vi "06c-arrays.vi"() -> ()   [LabVIEW 2018, in "LV2Julia_examples.lvlib"]
uses:
  LV2Julia_examples.lvlib
  LV2Julia_core/VIs/Server or client state.ctl
  statistics.ctl
  LV2Julia_core/VIs/Commands.ctl
  LV2Julia_core/VIs/ZMQ timeouts.ctl
  0d29fc62-3d1d-4713-a954-9c9e873b3633.vi
  aea790a6-a42b-4eb0-905f-734239196901.vi
  72a46192-383e-4ee5-9465-71670922b82a.vi
  ef5408d4-6538-41d1-b296-fda05a71e4b0.vi
  b8d67b76-17b0-4ad8-b521-2f6549c52c10.vi
  e4efb182-1b04-4d49-96a3-1defebd055ea.vi
  ef458cb0-9ca2-4aa9-bd1e-ad103f8bb0c0.vi
  9df197b6-2616-4b86-abf4-a70e9215d122.vi
  28751878-cf8c-4743-a8b0-c60d78ce5b36.vi
  c328879f-33e1-4261-a6aa-c93c9ebac265.vi
  0d29fc62-3d1d-4713-a954-9c9e873b3633.vi/8ee49078-a04b-40cf-aceb-de90d52f19ef.vi
  aea790a6-a42b-4eb0-905f-734239196901.vi/353007a7-a356-474a-8eac-0d4386ef6058.vi
  72a46192-383e-4ee5-9465-71670922b82a.vi/fff5125a-c1cf-426f-b211-502a59584787.vi
  ef5408d4-6538-41d1-b296-fda05a71e4b0.vi/38f70dbe-b881-407f-ae9e-ee3877922e21.vi
  b8d67b76-17b0-4ad8-b521-2f6549c52c10.vi/b12f13d0-0083-497f-bd73-45587d52367a.vi
  e4efb182-1b04-4d49-96a3-1defebd055ea.vi/02b7e865-0b9c-4fe2-9305-325b12209529.vi
  e4efb182-1b04-4d49-96a3-1defebd055ea.vi/bae9804c-4c06-4ca2-bba6-84ede4188db3.vi
  ef458cb0-9ca2-4aa9-bd1e-ad103f8bb0c0.vi/e8b90c0a-49a5-4093-b01b-c91da666bc06.vi
  9df197b6-2616-4b86-abf4-a70e9215d122.vi/e68dc8aa-e036-44d5-82eb-549111025a95.vi
  28751878-cf8c-4743-a8b0-c60d78ce5b36.vi/748d803b-9eab-4607-80f6-e121fa062447.vi
  c328879f-33e1-4261-a6aa-c93c9ebac265.vi/2931e3ef-e8d8-47e5-81f6-8bdf84f9b635.vi
  c328879f-33e1-4261-a6aa-c93c9ebac265.vi/2af4d478-d114-4323-a1a4-ea8d6e36c34a.vi
  72a46192-383e-4ee5-9465-71670922b82a.vi/fff5125a-c1cf-426f-b211-502a59584787.vi/7beb9e5a-56af-4202-a395-c072f8f6a12a.vi
  ef5408d4-6538-41d1-b296-fda05a71e4b0.vi/38f70dbe-b881-407f-ae9e-ee3877922e21.vi/706c9d30-0200-4f77-8390-edf6001941d7.vi
  b8d67b76-17b0-4ad8-b521-2f6549c52c10.vi/b12f13d0-0083-497f-bd73-45587d52367a.vi/c2cf4afe-14de-4a7c-a038-eb38a913b356.vi
  b8d67b76-17b0-4ad8-b521-2f6549c52c10.vi/b12f13d0-0083-497f-bd73-45587d52367a.vi/7452286d-6709-42b4-a933-263885f1ef29.vi
  b8d67b76-17b0-4ad8-b521-2f6549c52c10.vi/b12f13d0-0083-497f-bd73-45587d52367a.vi/11fbbbb9-4c5b-4442-95b0-52ac404484f0.vi
  e4efb182-1b04-4d49-96a3-1defebd055ea.vi/02b7e865-0b9c-4fe2-9305-325b12209529.vi/2a070854-1c7d-4d64-a736-cedc11a7f453.vi
  e4efb182-1b04-4d49-96a3-1defebd055ea.vi/02b7e865-0b9c-4fe2-9305-325b12209529.vi/ce6c50d9-0aec-4ce5-9563-f5a1f3a5f606.vi
  9df197b6-2616-4b86-abf4-a70e9215d122.vi/e68dc8aa-e036-44d5-82eb-549111025a95.vi/f53deb3e-8950-4786-9e71-9c0eddecade7.vi
  28751878-cf8c-4743-a8b0-c60d78ce5b36.vi/748d803b-9eab-4607-80f6-e121fa062447.vi/dbe84567-7ef4-485c-b551-38ee1d34b483.vi
  28751878-cf8c-4743-a8b0-c60d78ce5b36.vi/748d803b-9eab-4607-80f6-e121fa062447.vi/ee701064-8ef7-4cb3-acd2-d09a2ca746d4.vi
  28751878-cf8c-4743-a8b0-c60d78ce5b36.vi/748d803b-9eab-4607-80f6-e121fa062447.vi/44459596-931b-4795-b592-1aeed408307a.vi
  c328879f-33e1-4261-a6aa-c93c9ebac265.vi/2931e3ef-e8d8-47e5-81f6-8bdf84f9b635.vi/73e3ce9d-932f-4e3b-9fa0-1650b3f4c481.vi
  c328879f-33e1-4261-a6aa-c93c9ebac265.vi/2931e3ef-e8d8-47e5-81f6-8bdf84f9b635.vi/5f9fe6bb-1a1a-4cc4-87dc-92c210ea0b8d.vi
  72a46192-383e-4ee5-9465-71670922b82a.vi/fff5125a-c1cf-426f-b211-502a59584787.vi/7beb9e5a-56af-4202-a395-c072f8f6a12a.vi/02adab04-5a86-4a97-93e3-27cb657de44c.vi
  ef5408d4-6538-41d1-b296-fda05a71e4b0.vi/38f70dbe-b881-407f-ae9e-ee3877922e21.vi/706c9d30-0200-4f77-8390-edf6001941d7.vi/2e058e94-5032-4d2b-9353-3bd516f74917.vi
  e4efb182-1b04-4d49-96a3-1defebd055ea.vi/02b7e865-0b9c-4fe2-9305-325b12209529.vi/2a070854-1c7d-4d64-a736-cedc11a7f453.vi/5828844a-d6ce-4aa0-80c3-aaf83f58a5bd.vi
  9df197b6-2616-4b86-abf4-a70e9215d122.vi/e68dc8aa-e036-44d5-82eb-549111025a95.vi/f53deb3e-8950-4786-9e71-9c0eddecade7.vi/7afa4ec8-e56f-4750-a570-ce5d96af2d90.vi
  c328879f-33e1-4261-a6aa-c93c9ebac265.vi/2931e3ef-e8d8-47e5-81f6-8bdf84f9b635.vi/73e3ce9d-932f-4e3b-9fa0-1650b3f4c481.vi/979e58dc-c8d9-47e6-a478-8cf7a84a3445.vi
  LV2Julia_core/VIs/check ID validity.vi
  LV2Julia_core/VIs/bindata_descr to JSON.vi
  LV2Julia_core/VIs/check cluster field names.vi
  LV2Julia_core/VIs/concat JSON.vi
  LV2Julia_core/VIs/build request.vi
  LV2Julia_core/VIs/Parse server response.vi
  LV2Julia_core/VIs/log jl exceptions.vi
  <vilib>/Utility/error.llb/Error Cluster From Error Code.vi
  LV2Julia_core/LV2Julia_core.lvlib
panel:
  out "Statistics 1":T1={"size "=0, "mean"=nan, "median"=nan, "min"=nan, "max"=nan} caption="Statistics (ms)" {"min" format="%#.1f"; "max" format="%#.1f"; "median" format="%.1f"; "mean" format="%.1f"}
  in  "max size 1":i32=20 caption="sample max"
  out "Statistics 2":T1={"size "=0, "mean"=nan, "median"=nan, "min"=nan, "max"=nan} caption="Statistics (ms)" {"min" format="%#.1f"; "max" format="%#.1f"; "median" format="%.1f"; "mean" format="%.1f"}
  in  "max size 2":i32=20 caption="sample max"
  out "error info 2":string
  out "call duration (ms) 2":dbl format="%#.3f"
  in  "N - arr size 2":u16=4
  out "Input Matrix (NxN)2":dbl[][](array[numeric])=[[1.0, 0.0, 5.0], [4.0, 2.0, 1.0], [2.0, 2.0, 3.0]] format="%#.4g"
  in  "paus2":bool
  out "current error 2":errorcluster
  out "error info 1":string
  out "call duration (ms) 1":dbl format="%#.3f"
  in  "N - arr size 1":u16=4
  out "Solution Vector":dbl[](array[numeric]) format="%.4f"
  out "Known Vector":dbl[](array[numeric])=[22.0, 14.0, 18.0] format="%#.4g"
  out "Input Matrix (NxN) 1":dbl[][](array[numeric])=[[1.0, 0.0, 5.0], [4.0, 2.0, 1.0], [2.0, 2.0, 3.0]] format="%#.4g"
  in  "paus1":bool
  out "current error 1":errorcluster
  out "Eigenvalues":cdb[](array[numeric]) format="%.2f"
  out "final error":errorcluster
  in  "stop":bool
  out "ZMQ timeout":bool
  out "Jl Server state":T2
  # "Concurrent access to Julia server: Solving a system of linear equations in one loop, and computing eigenvalues in another one."
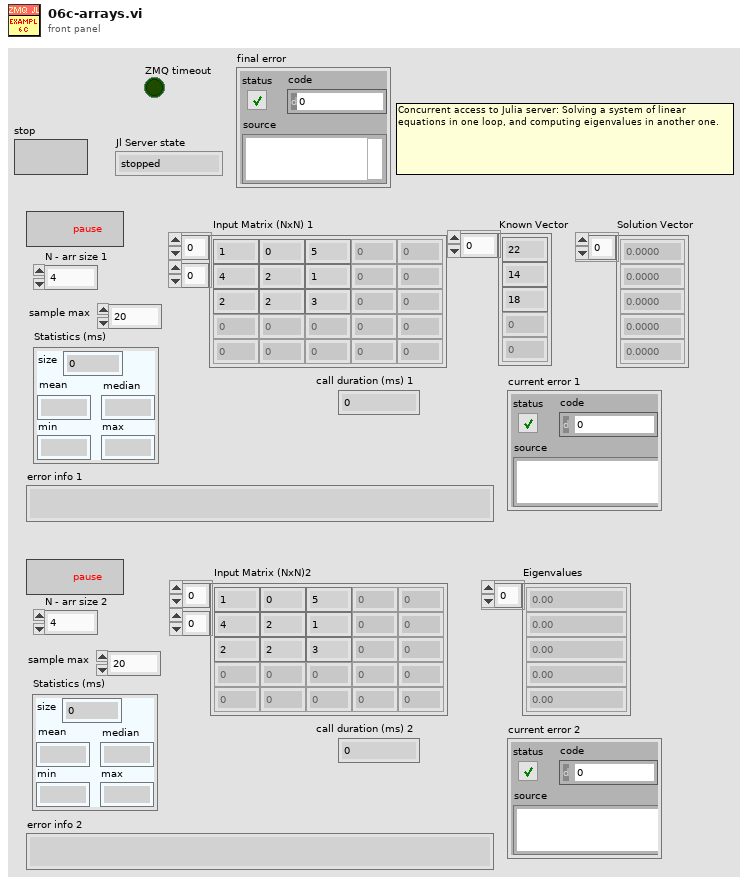
[diagram p1: front panel]
types:
  T1 = typedef "LV2Julia_examples.lvlib/statistics.ctl" = cluster{"size ":u32, "mean":dbl, "median":dbl, "min":dbl, "max":dbl}
  T2 = typedef "LV2Julia_core.lvlib/Server or client state.ctl" = enum16{"stopped", "running", "unknown"}
  T3 = typedef "LV2Julia_core.lvlib/ZMQ timeouts.ctl" = cluster{"SNDTIMEO":i32, "RCVTIMEO":i32}
  T4 = typedef "LV2Julia_core.lvlib/Commands.ctl" = enum16{"Start Jl-server & Init LV-client", "Send request & Get response ", "Stop Jl-server & Cleanup LV-client", "Cleanup LV-client", "Start Jl-server", "Stop Jl-server", "Init LV-Client", "Cleanup LV-Client", "(not allowed)", "Set LV Client state", "Set Jl Server state", "set ZMQ timeout", "read ZMQ timeout", "read-out state"}
  T5 = typedef "LV2Julia_core.lvlib/Bindata&description.ctl" = cluster{"bindata_descr":T6[], "bindata":u8[]}
  T6 = typedef "LV2Julia_core.lvlib/Bindata description.ctl" = cluster{"nofbytes":i32, "numtype":string, "start":i32, "arrdims":i32[], "kwarg_name":string, "category":string}
  T7 = typedef "LV2Julia_core.lvlib/detailed error info.ctl" = cluster{"exception_or_info":string, "trace":T8[]}
  T8 = typedef "LV2Julia_core.lvlib/StackFrame.ctl" = cluster{"frame_summary":string, "func":string, "linfo":string, "file":string, "line":i32, "pointer":u64, "from_c":bool, "inlined":bool}
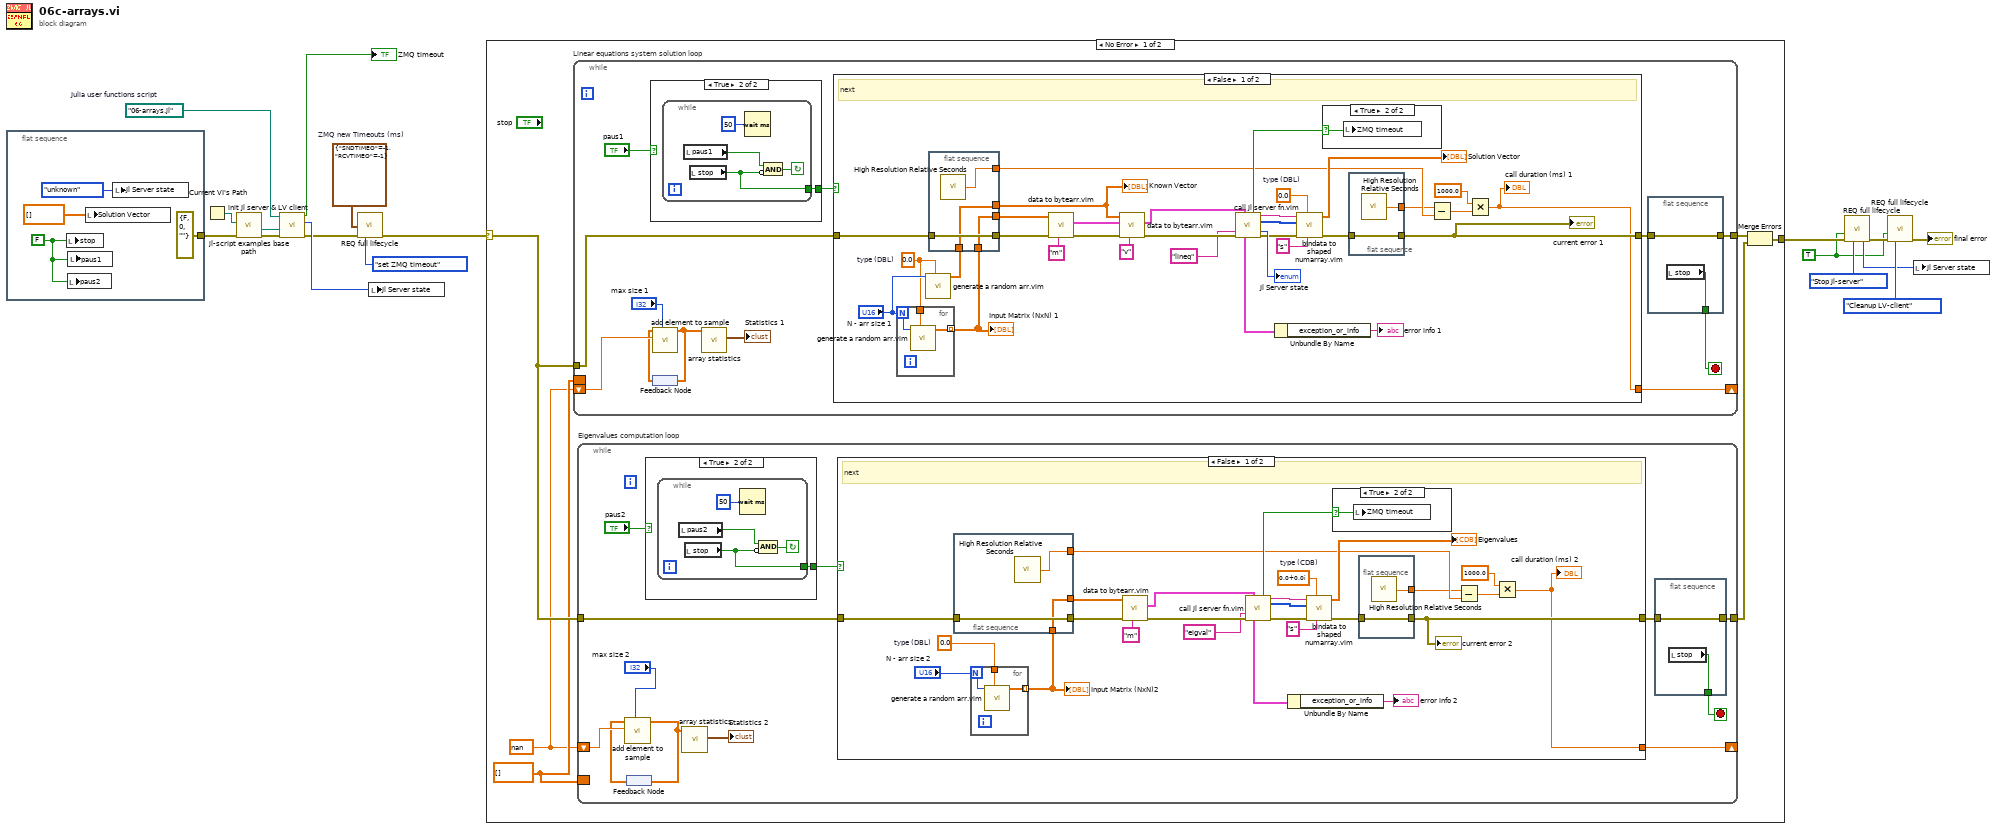
[diagram p0: block diagram]
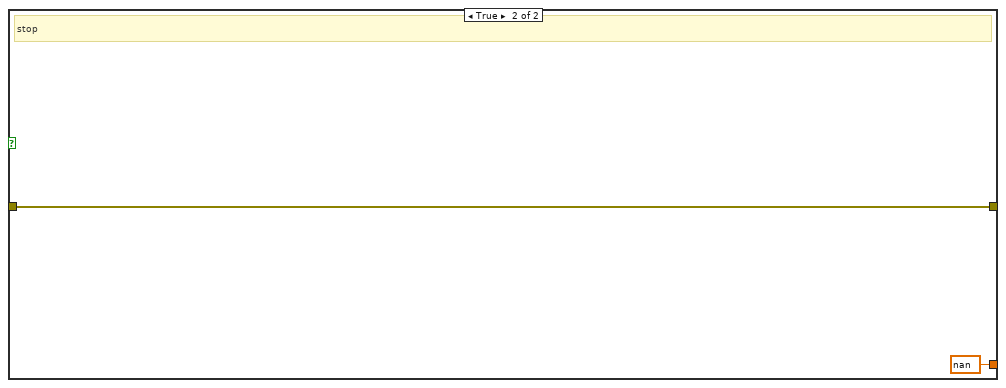
[diagram p4: hidden frame]
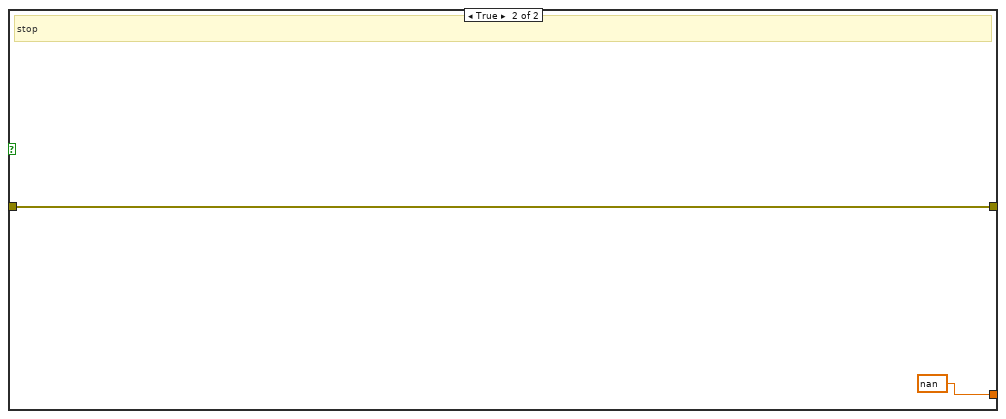
[diagram p7: hidden frame]
diagram:
  w9 = T3 {"SNDTIMEO"=-1, "RCVTIMEO"=-1}  # ZMQ new Timeouts (ms)
  w8 = path "06-arrays.jl"  # Julia user functions script
  w12 = TRUE ("Force command")
  n1 = flat-sequence {
    tunnel: [errorcluster {"status"=FALSE, "code"=0, "source"=""} ("error in (no error)")] -> w1
    frame #0 {
      w19 = FALSE ("stop")
      n2 = local write "stop"(w19) -> ()
      n3 = local write "paus2"(w19) -> ()
      n4 = local write "paus1"(w19) -> ()
      n5 = local write "Solution Vector"(dbl[] [] ("Server response")) -> ()
      n6 = local write "Jl Server state"(Server_or_client_state."unknown" ("Jl Server state out")) -> ()
    }
  }
  n7 = Current VI's Path() -> (path=w4:path)
  n8 = call "jl-script examples base path.vi"("error in (no error)"=w1, "calling example VI path"=w4) -> ("error out"=w3:errorcluster, "jl-script-examples base path"=w2:path)  [unwired: 8 in]
  n9 = call "init Jl server & LV client.vi"("error in (no error)"=w3, "Base path (not a path)"=w2, "Julia user functions script"=w8) -> ("error out"=w5:errorcluster, "Jl Server state out"=w6:T2, "timeout?"=→"ZMQ timeout":bool)  [unwired: 6 in]
  n10 = call "REQ full lifecycle.vi"("ZMQ new Timeouts in"=w9, "error in"=w5, "command"=Commands."set ZMQ timeout") -> ("error out"=w11:errorcluster)  [unwired: 6 in, 6 out]
  n11 = local write "Jl Server state"(w6) -> ()
  n12 = case shown="No Error" w11 {
    selector: w11 -> [w25 w148]
    tunnel: [w27 w148] -> w18
    frame No Error {
      w24 = dbl[] []
      w23 = nan
      n13 = while "Linear equations system solution loop" {
        tunnel: w25 -> [w91]
        tunnel: [w95] -> w28
        shift-right: [w90] -> _
        shift-left: w23 -> [w89]
        border: w24 -> [_]
        stop <- w94 stop-if-true
        n14 = case shown="True" "paus1" {
          tunnel: [_ w97] -> w93
          frame False {
          }
          frame True {
            n15 = while {
              tunnel: [w98] -> w97
              stop <- w99 continue-if-true
              n16 = local read "paus1"() -> (w100:bool)
              n17 = local read "stop"() -> (w98:bool)
              n18 = Wait (ms)(milliseconds to wait=u32 50) -> ()  [unwired: 1 out]
              n19 = Compound Arithmetic op=AND(w100, invert w98) -> (w99:bool)
            }
          }
        }
        n20 = feedback #1() -> (w87:dbl[])
        n21 = call "add element to sample.vi"("sample size in"="max size 1", "element in"=w89, "Array in"=w87) -> ("Array out"=w88:dbl[])  [unwired: 8 in]
        n22 = feedback-in #1(w88) -> ()
        n23 = call "array statistics.vi"("Array in"=w88) -> ("Statistics (ms)"=→"Statistics 1":T1)  [unwired: 10 in]
        n24 = case shown="False" w93 {
          tunnel: [w105 w147] -> w96
          tunnel: w91 -> [w120 w147]
          tunnel: [w104 nan] -> w90
          frame False {
            w129 = 0.0  # type (DBL)
            w132 = 0.0  # type (DBL)
            # "next"
            n25 = for {
              N: "N - arr size 1" -> [w142]
              tunnel: [w144] -> w112 mode=indexing
              tunnel: w129 -> [w143]
              n26 = call "generate a random arr.vim"("type in"=w143, "arr size"=w142) -> ("float out"=w144:dbl[])  [unwired: 5 in, 4 out]
            }
            "Input Matrix (NxN) 1" <- w112
            n27 = call "generate a random arr.vim"("type in"=w129, "arr size"="N - arr size 1") -> ("float out"=w117:dbl[])  [unwired: 5 in, 4 out]
            n28 = flat-sequence {
              tunnel: [w141] -> w119
              tunnel: w120 -> [w141]
              tunnel: w112 -> [w140]
              tunnel: [w140] -> w118
              tunnel: [w139] -> w107
              tunnel: w117 -> [w139]
              tunnel: [w138] -> w115
              frame #0 {
                n29 = call <vilib>:"High Resolution Relative Seconds.vi"() -> ("relative seconds"=w138:dbl)
              }
            }
            n30 = call "data to bytearr.vim"("kwarg_name"="m", "error in (no error)"=w119, "data in"=w118) -> ("error out"=w135:errorcluster, "Bindata & descr out"=w134:T5)  [unwired: 6 in, 1 out]
            n31 = call "data to bytearr.vim"("kwarg_name"="v", "error in (no error)"=w135, "Bindata & descr in"=w134, "data in"=w107) -> ("error out"=w121:errorcluster, "Bindata & descr out"=w125:T5)  [unwired: 5 in, 1 out]
            n32 = call "call Jl server fn.vim"("Bindata & descr in"=w125, "fun2call"="lineq" ("Julia function name"), "error in (no error)"=w121) -> ("timeout?"=w124:bool, "JSON received"=w123:string, "binary data received"=w122:u8[], "Jl Server state out"=→"Jl Server state":T2, "detailed error info"=w109:T7, "error out"=w126:errorcluster)  [unwired: 6 in, 1 out]
            n33 = Unbundle By Name(w109) -> ("exception_or_info"=→"error info 1":string)
            n34 = call "bindata to shaped numarray.vim"("name"="s" ("kwarg_name"), "element type"=w132, "error in (no error)"=w126, "binary data"=w122, "JSON in"=w123) -> ("error out"=w116:errorcluster, "numarray 1D"=→"Solution Vector":dbl[])  [unwired: 3 in, 2 out]
            n35 = case shown="True" w124 {
              selector: w124 -> [_ w145]
              frame False {
              }
              frame True {
                n36 = local write "ZMQ timeout"(w145) -> ()
              }
            }
            n37 = flat-sequence {
              tunnel: [w137] -> w105
              tunnel: w116 -> [w137]
              tunnel: [w136] -> w111
              frame #0 {
                n38 = call <vilib>:"High Resolution Relative Seconds.vi"() -> ("relative seconds"=w136:dbl)
              }
            }
            n39 = Subtract(x=w111, y=w115) -> (x-y=w114:dbl)
            n40 = Multiply(x=1000.0, y=w114) -> (x*y=w104:dbl)
            "call duration (ms) 1" <- w104
            "current error 1" <- w105
            "Known Vector" <- w107
          }
          frame True {
            # "stop"
          }
        }
        n41 = flat-sequence {
          tunnel: w96 -> [w103]
          tunnel: [w103] -> w95
          tunnel: [w102] -> w94
          frame #0 {
            n42 = local read "stop"() -> (w102:bool)
          }
        }
      }
      n43 = while "Eigenvalues computation loop" {
        tunnel: w25 -> [w40]
        tunnel: [w38] -> w26
        shift-right: [w34] -> _
        shift-left: w23 -> [w33]
        border: w24 -> [_]
        stop <- w37 stop-if-true
        n44 = feedback #2() -> (w30:dbl[])
        n45 = call "add element to sample.vi"("sample size in"="max size 2", "element in"=w33, "Array in"=w30) -> ("Array out"=w32:dbl[])  [unwired: 8 in]
        n46 = feedback-in #2(w32) -> ()
        n47 = case shown="True" "paus2" {
          tunnel: [_ w41] -> w36
          frame False {
          }
          frame True {
            n48 = while {
              tunnel: [w42] -> w41
              stop <- w43 continue-if-true
              n49 = local read "paus2"() -> (w44:bool)
              n50 = local read "stop"() -> (w42:bool)
              n51 = Wait (ms)(milliseconds to wait=u32 50) -> ()  [unwired: 1 out]
              n52 = Compound Arithmetic op=AND(w44, invert w42) -> (w43:bool)
            }
          }
        }
        n53 = call "array statistics.vi"("Array in"=w32) -> ("Statistics (ms)"=→"Statistics 2":T1)  [unwired: 10 in]
        n54 = case shown="False" w36 {
          tunnel: [w51 w84] -> w39
          tunnel: w40 -> [w62 w84]
          tunnel: [w48 nan] -> w34
          frame False {
            w70 = 0.0  # type (DBL)
            w72 = cdb 0.0+0.0i  # type (CDB)
            # "next"
            n55 = flat-sequence {
              tunnel: [w78] -> w61
              tunnel: w62 -> [w78]
              tunnel: w52 -> [w77]
              tunnel: [w77] -> w60
              tunnel: [w76] -> w58
              frame #0 {
                n56 = call <vilib>:"High Resolution Relative Seconds.vi"() -> ("relative seconds"=w76:dbl)
              }
            }
            n57 = for {
              N: "N - arr size 2" -> [w79]
              tunnel: [w81] -> w52 mode=indexing
              tunnel: w70 -> [w80]
              n58 = call "generate a random arr.vim"("type in"=w80, "arr size"=w79) -> ("float out"=w81:dbl[])  [unwired: 5 in, 4 out]
            }
            "Input Matrix (NxN)2" <- w52
            n59 = call "data to bytearr.vim"("kwarg_name"="m", "error in (no error)"=w61, "data in"=w60) -> ("error out"=w63:errorcluster, "Bindata & descr out"=w67:T5)  [unwired: 6 in, 1 out]
            n60 = call "call Jl server fn.vim"("Bindata & descr in"=w67, "fun2call"="eigval" ("Julia function name"), "error in (no error)"=w63) -> ("timeout?"=w66:bool, "JSON received"=w65:string, "binary data received"=w64:u8[], "detailed error info"=w53:T7, "error out"=w68:errorcluster)  [unwired: 6 in, 2 out]
            n61 = Unbundle By Name(w53) -> ("exception_or_info"=→"error info 2":string)
            n62 = call "bindata to shaped numarray.vim"("name"="s" ("kwarg_name"), "element type"=w72, "error in (no error)"=w68, "binary data"=w64, "JSON in"=w65) -> ("error out"=w59:errorcluster, "numarray 1D"=→"Eigenvalues":cdb[])  [unwired: 3 in, 2 out]
            n63 = case shown="True" w66 {
              selector: w66 -> [_ w82]
              frame False {
              }
              frame True {
                n64 = local write "ZMQ timeout"(w82) -> ()
              }
            }
            n65 = flat-sequence {
              tunnel: [w75] -> w51
              tunnel: w59 -> [w75]
              tunnel: [w74] -> w55
              frame #0 {
                n66 = call <vilib>:"High Resolution Relative Seconds.vi"() -> ("relative seconds"=w74:dbl)
              }
            }
            n67 = Subtract(x=w55, y=w58) -> (x-y=w57:dbl)
            n68 = Multiply(x=1000.0, y=w57) -> (x*y=w48:dbl)
            "call duration (ms) 2" <- w48
            "current error 2" <- w51
          }
          frame True {
            # "stop"
          }
        }
        n69 = flat-sequence {
          tunnel: w39 -> [w47]
          tunnel: [w47] -> w38
          tunnel: [w46] -> w37
          frame #0 {
            n70 = local read "stop"() -> (w46:bool)
          }
        }
      }
      n71 = Merge Errors(w28, w26) -> (w27:errorcluster)
    }
    frame Error {
    }
  }
  n72 = call "REQ full lifecycle.vi"("Force command"=w12, "error in"=w18, "command"=Commands."Stop Jl-server") -> ("Jl Server state out"=w13:T2, "error out"=w16:errorcluster)  [unwired: 6 in, 5 out]
  n73 = call "REQ full lifecycle.vi"("Force command"=w12, "error in"=w16, "command"=Commands."Cleanup LV-client") -> ("error out"=→"final error":errorcluster)  [unwired: 6 in, 6 out]
  n74 = local write "Jl Server state"(w13) -> ()
